vi "lm Color Enable.vi"(8 "error in (no error)":errorcluster, 10 "str_State":string, 11 "str_Color":string) -> (0 "error out":errorcluster, 2 "str_State out":string, 3 "str_Color out":string)   [LabVIEW 2017, in "LumencorDLLDbg64.lvlib"]
doc: "The Color Enable function will turn the selected color ON or OFF.\n\n\n\n\nextern \"C\" LUMENCORDLL2B_API void lmColorEnable(char *str_Color, char *str_State);"
uses:
  LumencorDLLDbg64.lvlib
  LumencorDLLDbg64.dll
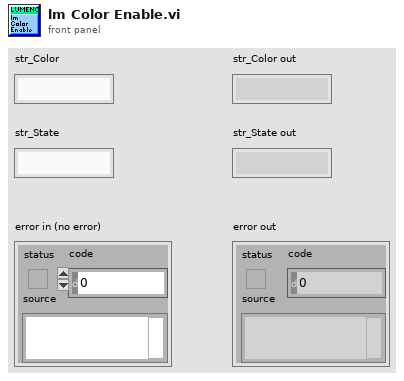
[diagram p1: front panel]
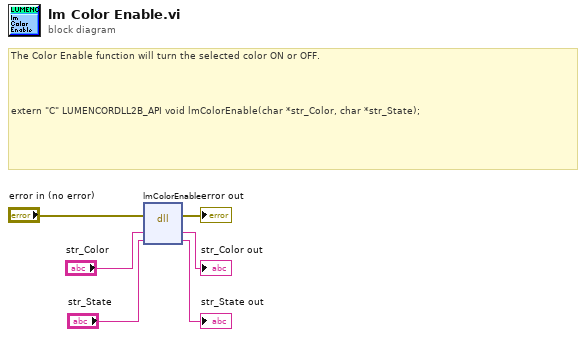
[diagram p0: block diagram]
diagram:
  # "The Color Enable function will turn the selected color ON or OFF.\n\n\n\n\nextern \"C\" LUMENCORDLL2B_API void lmColorEnable(char *str_Color, char *str_State);"
  n1 = dll-call lib="Q:/GIT -- Lumencor DLL4/LabVIEW Library (64bit)/LumencorDLLDbg64.*" fn="lmColorEnable"(error in="error in (no error)", "str_Color"="str_Color", "str_State"="str_State") -> (error out=→"error out":errorcluster, "str_Color"=→"str_Color out":string, "str_State"=→"str_State out":string)  [unwired: 3 in, 1 out]
